vi "GenerateControlList.vi"(11 "ListType":string) -> (3 "ControlList":string[](array[string]))   [LabVIEW 2016, in "M1M3SupportEUI_Views.lvlib"]
uses:
  M1M3SupportEUI_Views.lvlib
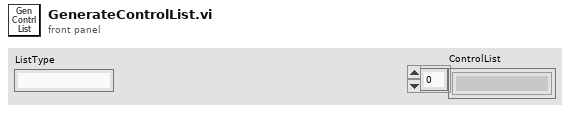
[diagram p1: front panel]
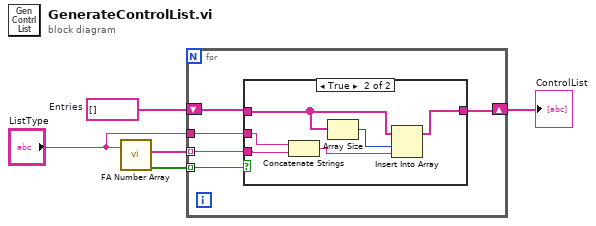
[diagram p0: block diagram]
diagram:
  w5 = string[] []  # Entries
  n1 = call "FA Number Array.vi"("Data Type"="ListType") -> ("On/Off Array"=w2:bool[], "FA Number String Array"=w3:string[])  [unwired: 8 in, 1 out]
  n2 = for {
    shift-right: [w9] -> w4
    shift-left: w5 -> [w10]
    tunnel: w3 -> [w8] mode=indexing
    tunnel: w2 -> [w7] mode=indexing
    tunnel: "ListType" -> [w6]
    n3 = case shown="True" w7 {
      tunnel: w8 -> [_ w17]
      tunnel: w10 -> [w11 w16]
      tunnel: [w11 w13] -> w9
      tunnel: w6 -> [_ w12]
      frame False {
      }
      frame True {
        n4 = Concatenate Strings(w12, w17) -> (w14:string)
        n5 = Array Size(array=w16) -> (size(s)=w15:i32)
        n6 = Insert Into Array(array=w16, index=w15, new element=w14) -> (w13:string[])
      }
    }
  }
  "ControlList" <- w4
